vi "EEGstats(subvi).vi"(5 "Vstupní EEG":waveform(dbl)) -> (0 "Beta vlny":waveform(dbl), 1 "Alpha vlny":waveform(dbl), 2 "Theta vlny":waveform(dbl), 3 "Delta vlny":waveform(dbl))   [LabVIEW 2026]
uses:
  <vilib>/Analysis/3filter.llb/Filter Passband Type.ctl
  <vilib>/Analysis/3filter.llb/Butterworth Filter (DBL).vi
  <vilib>/Analysis/NI_AALBase.lvlib
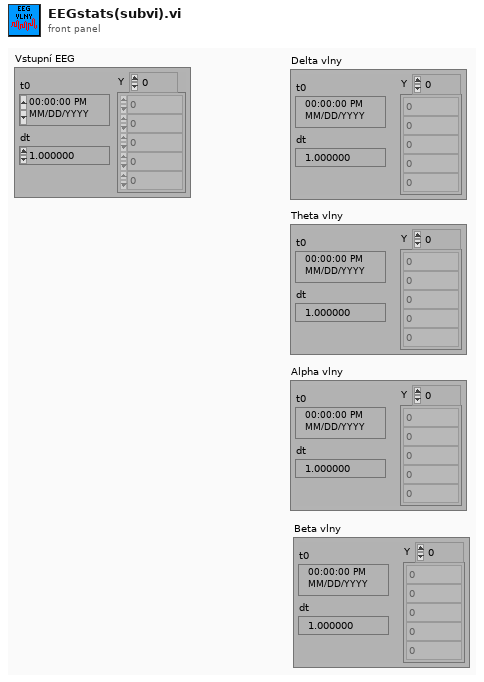
[diagram p1: front panel]
types:
  T1 = typedef "NI_AALBase.lvlib/Filter Passband Type.ctl" = enum32{"Lowpass", "Highpass", "Bandpass", "Bandstop"}
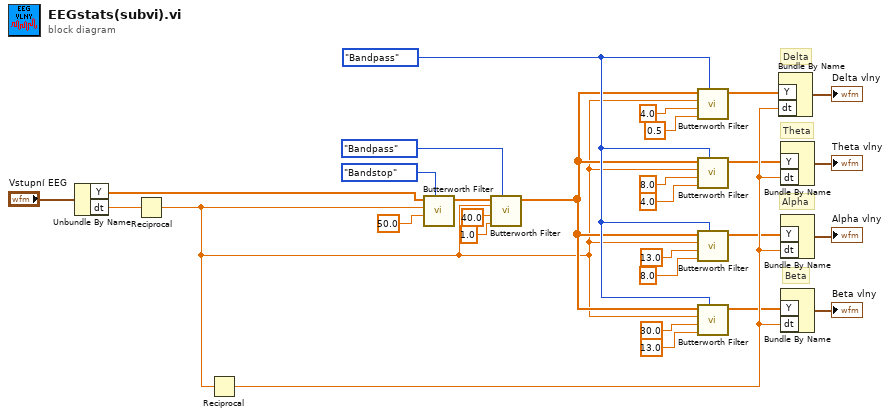
[diagram p0: block diagram]
diagram:
  w25 = Filter_Passband_Type."Bandpass" ("filter type")
  # "Beta"
  # "Alpha"
  # "Theta"
  # "Delta"
  n1 = Unbundle By Name("Vstupní EEG") -> ("Y"=w2:dbl[], "dt"=w4:dbl)
  n2 = Reciprocal(x=w4) -> (1/x=w1:dbl)
  n3 = Reciprocal(x=w1) -> (1/x=w16:dbl)
  n4 = call-poly <vilib>:"Butterworth Filter.vi"("filter type"=Filter_Passband_Type."Bandstop", "high cutoff freq: fh"=50.0, "sampling freq: fs"=w1, "X"=w2) -> ("Filtered X"=w11:dbl[])  [unwired: 4 in, 1 out]
  n5 = call-poly <vilib>:"Butterworth Filter.vi"("filter type"=Filter_Passband_Type."Bandpass", "low cutoff freq: fl"=1.0, "high cutoff freq: fh"=40.0, "sampling freq: fs"=w1, "X"=w11) -> ("Filtered X"=w5:dbl[])  [unwired: 3 in, 1 out]
  n6 = call-poly <vilib>:"Butterworth Filter.vi"("filter type"=w25, "low cutoff freq: fl"=0.5, "high cutoff freq: fh"=4.0, "sampling freq: fs"=w1, "X"=w5) -> ("Filtered X"=w12:dbl[])  [unwired: 3 in, 1 out]
  n7 = call-poly <vilib>:"Butterworth Filter.vi"("filter type"=w25, "low cutoff freq: fl"=4.0, "high cutoff freq: fh"=8.0, "sampling freq: fs"=w1, "X"=w5) -> ("Filtered X"=w15:dbl[])  [unwired: 3 in, 1 out]
  n8 = call-poly <vilib>:"Butterworth Filter.vi"("filter type"=w25, "low cutoff freq: fl"=8.0, "high cutoff freq: fh"=13.0, "sampling freq: fs"=w1, "X"=w5) -> ("Filtered X"=w14:dbl[])  [unwired: 3 in, 1 out]
  n9 = call-poly <vilib>:"Butterworth Filter.vi"("filter type"=w25, "low cutoff freq: fl"=13.0, "high cutoff freq: fh"=30.0, "sampling freq: fs"=w1, "X"=w5) -> ("Filtered X"=w13:dbl[])  [unwired: 3 in, 1 out]
  n10 = Bundle By Name("Y"=w12, "dt"=w16) -> (→"Delta vlny":waveform(dbl))  [unwired: 1 in]
  n11 = Bundle By Name("Y"=w15, "dt"=w16) -> (→"Theta vlny":waveform(dbl))  [unwired: 1 in]
  n12 = Bundle By Name("Y"=w14, "dt"=w16) -> (→"Alpha vlny":waveform(dbl))  [unwired: 1 in]
  n13 = Bundle By Name("Y"=w13, "dt"=w16) -> (→"Beta vlny":waveform(dbl))  [unwired: 1 in]
